vi "Stock html index.vi"(7 "Under Construction":bool[](array[boolean]), 10 "Mathcad version":i32, 11 "Method":T1) -> (3 "HTML":string)   [LabVIEW 2012]
uses:
  Method.ctl
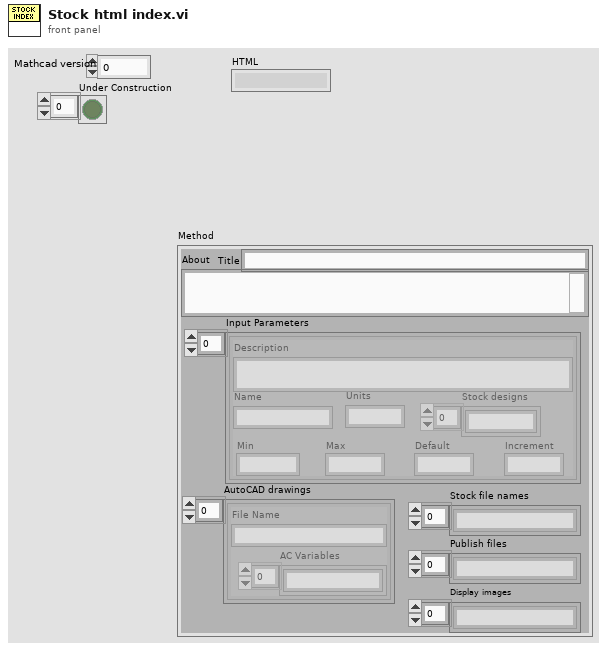
[diagram p1: front panel]
types:
  T1 = typedef "Method.ctl" = cluster{"Title":string, "About":string, "Input Parameters":cluster{"Description":string, "Name":string, "Min":string, "Max":string, "Default":string, "Units":string, "Increment":string, "Stock designs":string[]}[], "AutoCAD drawings":cluster{"File Name":string, "AC Variables":string[]}[], "Stock file names":string[], "Publish files":string[], "Display images":string[]}
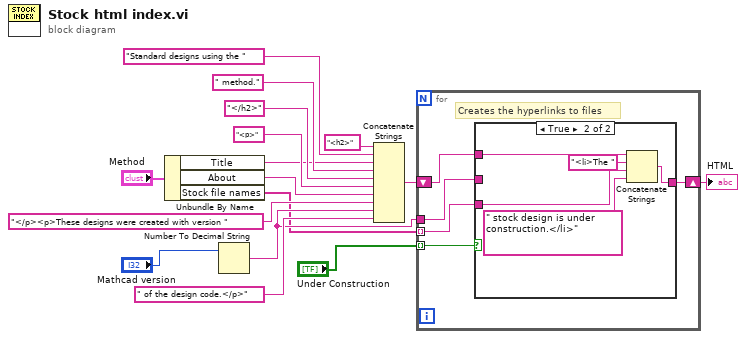
[diagram p0: block diagram]
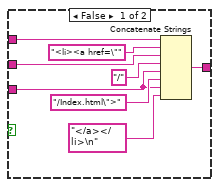
[diagram p2: hidden frame]
diagram:
  n1 = Unbundle By Name("Method") -> ("Title"=w4:string, "About"=w5:string, "Stock file names"=w3:string[])
  n2 = Number To Decimal String(number="Mathcad version") -> (decimal integer string=w15:string)  [unwired: 1 in]
  n3 = Concatenate Strings("<h2>" ("string"), "Standard designs using the " ("string"), w4, " method." ("string"), "</h2>" ("string"), "<p>" ("string"), w5, "</p><p>These designs were created with version " ("string"), w15, " of the design code.</p>" ("string")) -> (w11:string)
  n4 = for {
    shift-right: [w20] -> w2
    shift-left: w11 -> [w21]
    tunnel: w3 -> [w18] mode=indexing
    tunnel: w15 -> [w19]
    tunnel: "Under Construction" -> [w17] mode=indexing
    # "Creates the hyperlinks to files"
    n5 = case shown="True" w17 {
      tunnel: w21 -> [w26 w34]
      tunnel: [w25 w33] -> w20
      tunnel: w19 -> [w24 _]
      tunnel: w18 -> [w22 w32]
      frame False {
        n6 = Concatenate Strings(w26, "<li><a href=\"" ("string"), w24, "/" ("string"), w22, "/Index.html\">" ("string"), w22, "</a></li>\n" ("string")) -> (w25:string)
      }
      frame True {
        n7 = Concatenate Strings(w34, "<li>The " ("string"), w32, " stock design is under construction.</li>" ("string")) -> (w33:string)
      }
    }
  }
  "HTML" <- w2
